vi "Insert Word Into Little-Endian Bytes Poly.vi"   [LabVIEW 2020, in "NI_Bit Manipulation.lvlib"]
doc: "Convert an integer to a byte array in network byte order, i.e., big-endian. This polymorphic VI wraps an underlying malleable VI."
uses:
  <vilib>/Bit Manipulation/NI_Bit Manipulation.lvlib
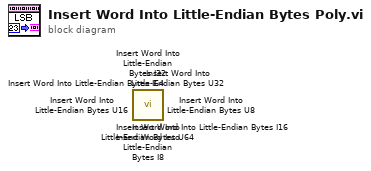
[diagram p0: block diagram]
diagram:
  n1 = call <vilib>:"Insert Word Into Little-Endian Bytes U64.vi"() -> ()  [unwired: 10 in, 2 out]
  n2 = call <vilib>:"Insert Word Into Little-Endian Bytes U32.vi"() -> ()  [unwired: 10 in, 2 out]
  n3 = call <vilib>:"Insert Word Into Little-Endian Bytes U16.vi"() -> ()  [unwired: 10 in, 2 out]
  n4 = call <vilib>:"Insert Word Into Little-Endian Bytes U8.vi"() -> ()  [unwired: 10 in, 2 out]
  n5 = call <vilib>:"Insert Word Into Little-Endian Bytes I64.vi"() -> ()  [unwired: 10 in, 2 out]
  n6 = call <vilib>:"Insert Word Into Little-Endian Bytes I32.vi"() -> ()  [unwired: 10 in, 2 out]
  n7 = call <vilib>:"Insert Word Into Little-Endian Bytes I16.vi"() -> ()  [unwired: 10 in, 2 out]
  n8 = call <vilib>:"Insert Word Into Little-Endian Bytes I8.vi"() -> ()  [unwired: 10 in, 2 out]
